vi "WPI_DashboardUpdate Command Params.vi"(8 "Update":bool=TRUE, 9 "NewVal":i32, 10 "Commands":string[][](array[string]), 11 "Param Tbl":refnum<vi>) -> (2 "params":i32)   [LabVIEW 2017]
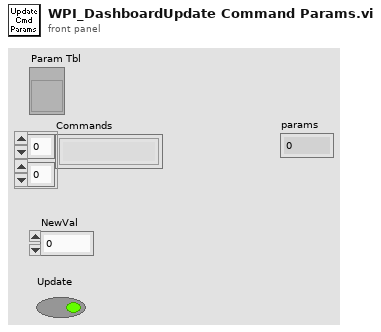
[diagram p1: front panel]
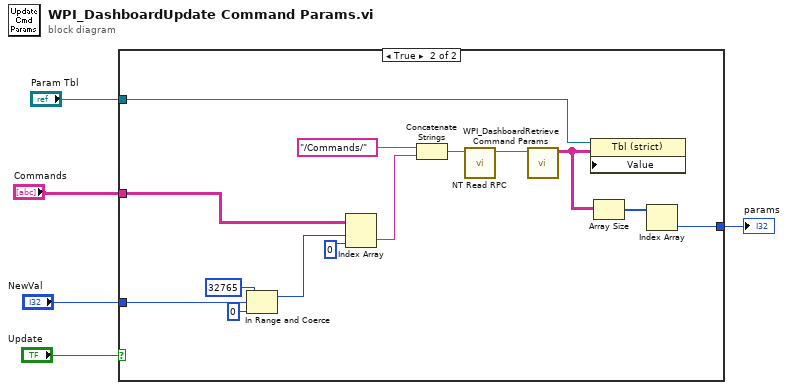
[diagram p0: block diagram]
diagram:
  n1 = case shown="True" "Update" {
    tunnel: "Param Tbl" -> [_ w14]
    tunnel: "Commands" -> [_ w9]
    tunnel: "NewVal" -> [_ w11]
    tunnel: [_ w6] -> w1
    frame False {
    }
    frame True {
      n2 = In Range and Coerce(upper limit=32765, x=w11, lower limit=0) -> (coerced(x)=w10:i32)  [unwired: 1 out]
      n3 = Index Array(array=w9, index (row)=w10, index (col)=0) -> (element=w19:string)
      n4 = Concatenate Strings("/Commands/", w19) -> (w16:string)
      n5 = call <vilib>:"NT Read RPC.vi"("Name"=w16) -> ("RPC Buffer"=w15:string)  [unwired: 9 in, 1 out]
      n6 = call <vilib>:"WPI_DashboardRetrieve Command Params.vi"("RPC Buffer"=w15) -> ("Param Info"=w8:string[][])  [unwired: 10 in]
      n7 = property class="Tbl (strict)"(reference=w14, "Value"=w8) -> ()  [unwired: 1 in, 2 out]
      n8 = Array Size(array=w8) -> (size(s)=w7:i32[])
      n9 = Index Array(array=w7) -> (element=w6:i32)  [unwired: 1 in]
    }
  }
  "params" <- w1
